vi "IMAQ crop image.vi"(0 "Image":T1, 1 "Square Image Size":i32=300) -> (7 "Cropped":T1(plugin-control))   [LabVIEW 2012, in "LightPipes.lvlib"]
uses:
  LightPipes.lvlib
  <vilib>/vision/Image Controls.llb/IMAQ Image.ctl
  <vilib>/vision/NI_Vision_Development_Module.lvlib
panel:
  out "Crop Rectangle":dbl[](array[numeric])
  out "Origin":T1(plugin-control)
  out "Centroid":cluster{"X Centroid":sgl, "Y Centroid":sgl} {"Y Centroid" format="%.2f"; "X Centroid" format="%.2f"}
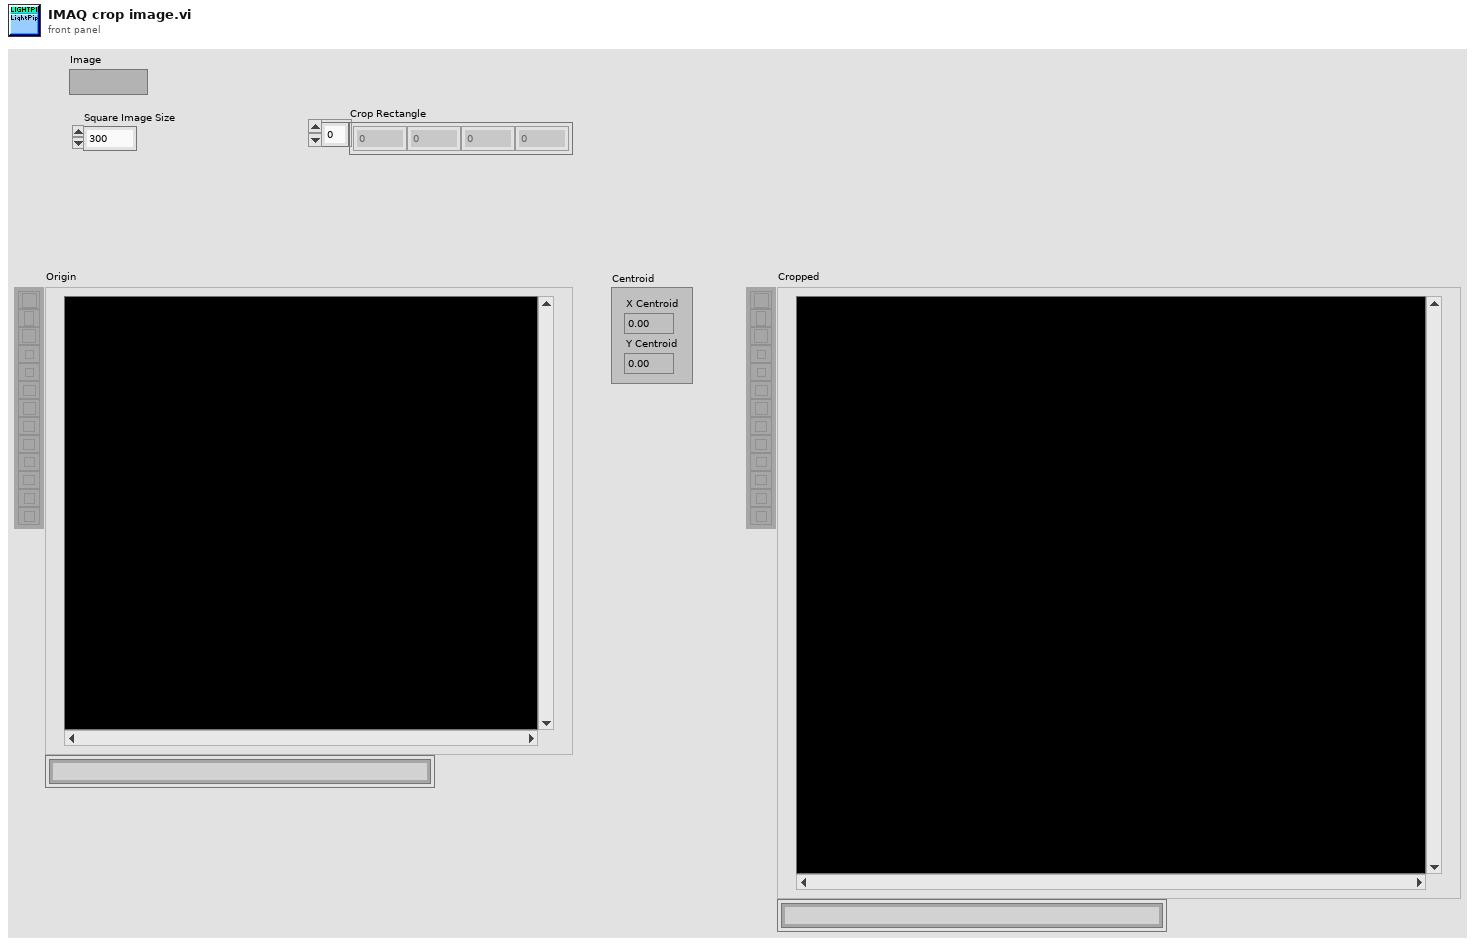
[diagram p1: front panel]
types:
  T1 = typedef "IMAQ Image.ctl" = refnum<image>
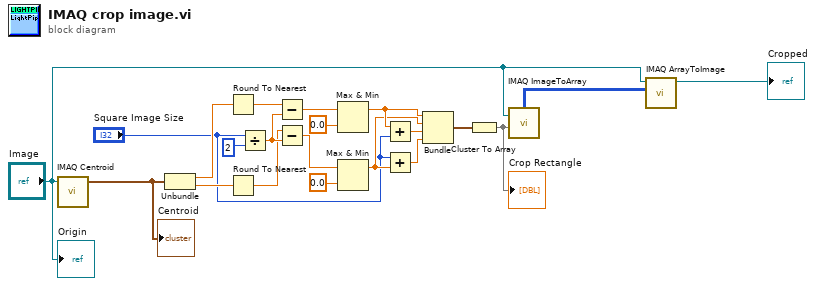
[diagram p0: block diagram]
diagram:
  n1 = call "IMAQ Centroid"("Image"="Image") -> ("Centroid"=w19:cluster{"X Centroid":sgl, "Y Centroid":sgl})  [unwired: 3 in, 1 out]
  "Centroid" <- w19
  n2 = Unbundle(w19) -> ("X Centroid"=w18:sgl, "Y Centroid"=w17:sgl)
  n3 = Round To Nearest(number=w18) -> (nearest integer value=w11:sgl)
  n4 = Round To Nearest(number=w17) -> (nearest integer value=w10:sgl)
  n5 = Divide(x="Square Image Size", y=2) -> (x/y=w12:dbl)
  n6 = Subtract(x=w11, y=w12) -> (x-y=w16:dbl)
  n7 = Subtract(x=w10, y=w12) -> (x-y=w14:dbl)
  n8 = Max & Min(x=w16, y=0.0) -> (max(x,y)=w6:dbl)  [unwired: 1 out]
  n9 = Max & Min(x=w14, y=0.0) -> (max(x,y)=w4:dbl)  [unwired: 1 out]
  n10 = Add(x=w6, y="Square Image Size") -> (x+y=w5:dbl)
  n11 = Add(x="Square Image Size", y=w4) -> (x+y=w2:dbl)
  n12 = Bundle "Bundle"(w6, w4, w5, w2) -> (w7:cluster{dbl, dbl, dbl, dbl})  [unwired: 1 in]
  n13 = Cluster To Array(cluster=w7) -> (array=w8:dbl[])
  "Crop Rectangle" <- w8
  n14 = call "IMAQ ImageToArray"("Optional Rectangle"=w8, "Image"="Image") -> ("Image Pixels (U8)"=w9:u8[][])  [unwired: 2 in, 4 out]
  n15 = call "IMAQ ArrayToImage"("Image Pixels (U8)"=w9, "Image"="Image") -> ("Image Out"=→"Cropped":T1)  [unwired: 8 in, 1 out]
  "Origin" <- "Image"
